vi "Get Gyro ID.vi"(2 "APDM Context":T1={"APDM Context ID"=0, "Gyro Mode"="", "Log Data"=FALSE, "Log File"=refnum, "Gyro Record Log"=refnum, "Gyro CMD Log"=refnum, "L Opal SN"=0, "R Opal SN"=0, "Access Point ID"=0, "Left Gyro Sim Data"=path "C:/Users/jfalesi/Desktop/CP FES Walking Code/Original/Ahad Vi/CP Code/Offline data/TD_7_Raw_R.txt", "Right Gyro Sim Data"=path "C:/Users/jfalesi/Desktop/CP FES Walking Code/Original/Ahad Vi/CP Code/Offline data/TD_7_Raw_R.txt", "Sampling Rate"=0.0, "Gyro Sim Time Array"=[], "Missed Gyro Count"=0.0}, 3 "Left or Right":T2) -> (0 "Opal SN":dbl, 1 "L or R":string)   [LabVIEW 2019]
uses:
  Archive/CP_FES_Walking_w_stim_on_off.llb/Left_Right_Control.ctl
  Controls/APDM Context Cluster.ctl
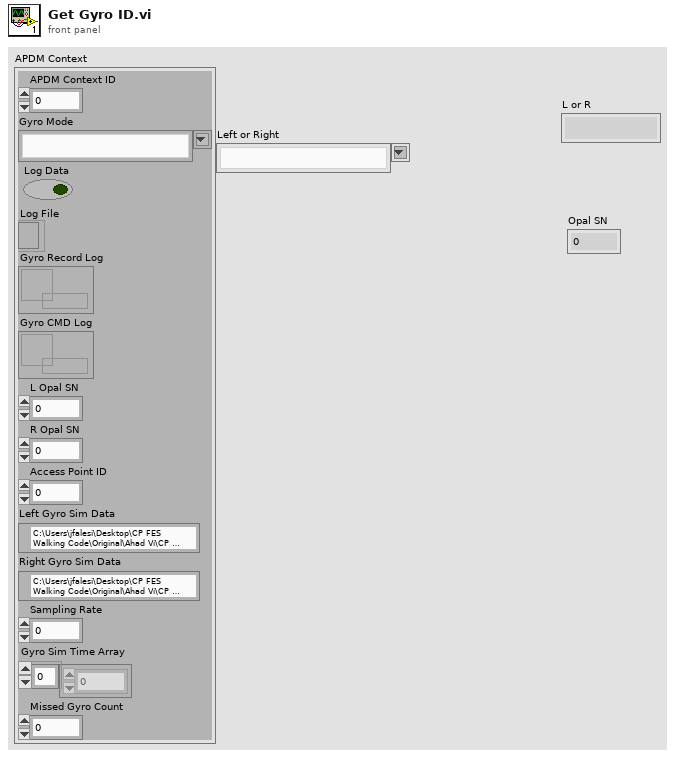
[diagram p1: front panel]
types:
  T1 = typedef "APDM Context Cluster.ctl" = cluster{"APDM Context ID":u32, "Gyro Mode":string, "Log Data":bool, "Log File":refnum<file>, "Gyro Record Log":refnum<queue>, "Gyro CMD Log":refnum<queue>, "L Opal SN":u32, "R Opal SN":u32, "Access Point ID":u32, "Left Gyro Sim Data":path, "Right Gyro Sim Data":path, "Sampling Rate":dbl, "Gyro Sim Time Array":dbl[], "Missed Gyro Count":dbl}
  T2 = typedef "Left_Right_Control.ctl" = string
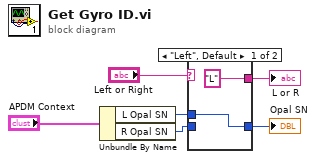
[diagram p0: block diagram]
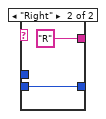
[diagram p2: hidden frame]
diagram:
  n1 = Unbundle By Name("APDM Context") -> ("L Opal SN"=w3:u32, "R Opal SN"=w2:u32)
  n2 = case shown="\"Left\", Default" "Left or Right" {
    tunnel: w3 -> [w8 _]
    tunnel: w2 -> [_ w10]
    tunnel: [w8 w10] -> w6
    tunnel: ["L" "R"] -> w4
    frame "Left", Default {
    }
    frame "Right" {
    }
  }
  "Opal SN" <- w6
  "L or R" <- w4
